vi "Model Initial Values - Main On Save Action.vi"(8 "error in (no error)":errorcluster, 11 "Device Item Ref in":T1 format="%.0x") -> (0 "error out":errorcluster, 3 "Device Item Ref out":T1 format="%.0x")   [LabVIEW 2011, in "Model Initial Values Custom Device.lvlib"]
uses:
  Model Initial Values Custom Device.lvlib
  <vilib>/NI Veristand/Custom Device API/Custom Device Item Ref.ctl
  Model Initial Values - Global.vi
  <vilib>/NI Veristand/Custom Device API/Custom Device API.lvlib
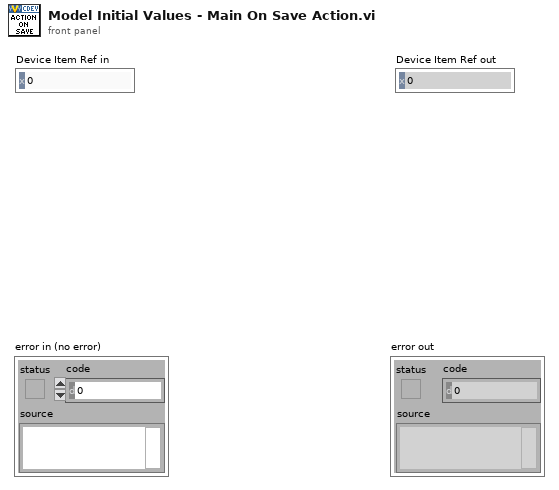
[diagram p1: front panel]
types:
  T1 = typedef "Custom Device API.lvlib/Custom Device Item Ref.ctl" = u64
  T2 = cluster{"Name":string, "Is Channel":bool, "GUID":string}
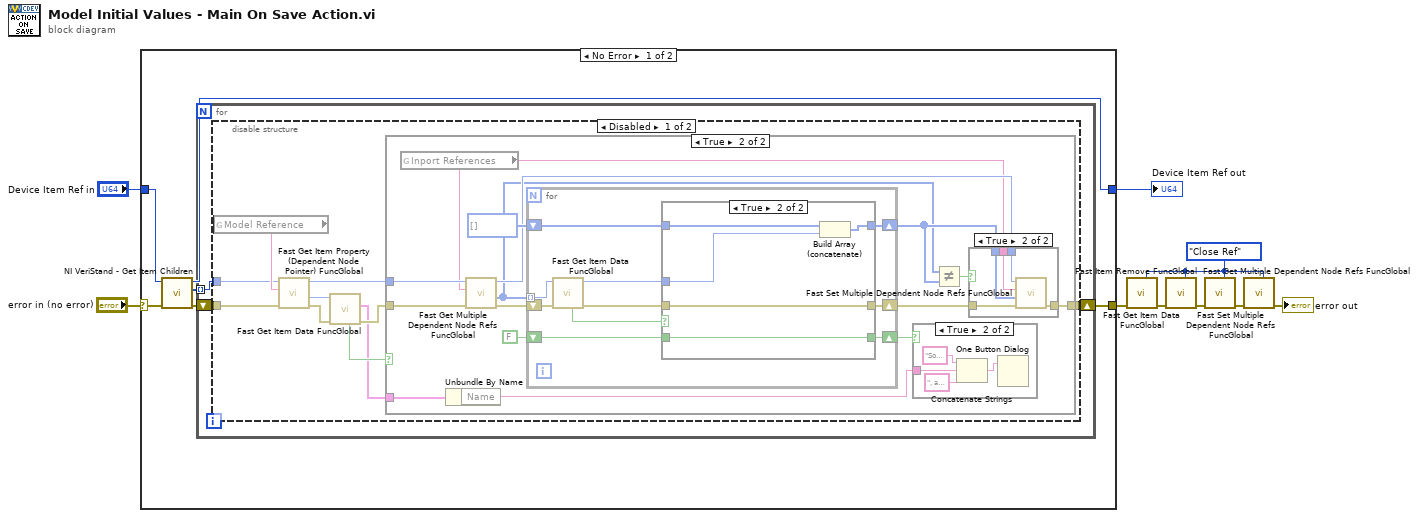
[diagram p0: block diagram]
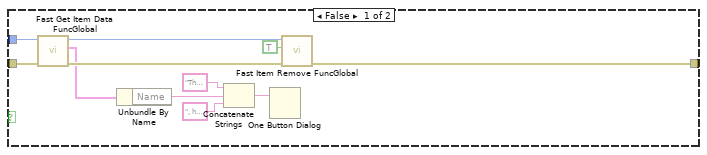
[diagram p2: hidden frame]
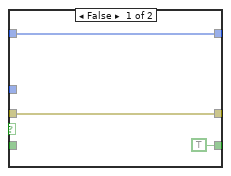
[diagram p5: hidden frame]
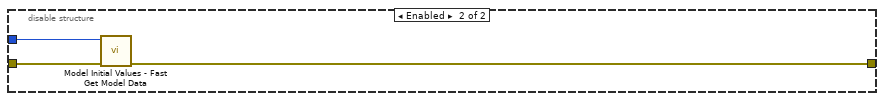
[diagram p6: hidden frame]
diagram:
  w1 = enum16{"Open or Add", "Close Ref"}."Close Ref" ("Action")
  n1 = case shown="No Error" "error in (no error)" {
    selector: "error in (no error)" -> [w14 w87]
    tunnel: [w15 w87] -> w6
    tunnel: "Device Item Ref in" -> [w12 w86]
    tunnel: [w10 w86] -> w7
    frame No Error {
      n2 = call <vilib>:"NI VeriStand - Get Item Children.vi"("error in (no error)"=w14, "Item Ref in"=w12) -> ("error out"=w13:errorcluster, "Child Refs"=w11:T1[], "Item Ref out"=w10:T1)  [unwired: 6 in, 1 out]
      n3 = for {
        shift-right: [w18] -> w15
        shift-left: w13 -> [w17]
        tunnel: w11 -> [w16] mode=indexing
        n4 = disable-structure shown="Disabled" {
          disable-tunnel: [w21 w83] -> w18
          disable-tunnel: w17 -> [w20 w85]
          disable-tunnel: w16 -> [w19 w84]
          frame Disabled {
            # "Initialization code."
            n5 = global read "Model Initial Values - Global.vi" "Model Reference"() -> (w23:string)
            n6 = call "Fast Get Item Property (Dependent Node Pointer) FuncGlobal.vi"("error in (no error)"=w20, "Property Name"=w23, "Item Ref in"=w19) -> ("error out"=w24:errorcluster, "Dependent Node Ref"=w26:T1, "Item Ref out"=w28:T1)  [unwired: 5 in, 1 out]
            n7 = call "Fast Get Item Data FuncGlobal.vi"("error in (no error)"=w24, "Item Ref in"=w26) -> ("error out"=w25:errorcluster, "Item Info"=w22:T2, "Found"=w27:bool)  [unwired: 6 in, 1 out]
            n8 = case shown="True" w27 {
              tunnel: [w34 w47] -> w21
              tunnel: w28 -> [w32 w53]
              tunnel: w25 -> [w33 w52]
              tunnel: w22 -> [_ w44]
              frame False {
                n9 = call "Fast Get Item Data FuncGlobal.vi"("error in (no error)"=w33, "Item Ref in"=w32) -> ("error out"=w30:errorcluster, "Item Info"=w29:T2, "Item Ref out"=w31:T1)  [unwired: 6 in, 1 out]
                n10 = Unbundle By Name(w29) -> ("Name"=w35:string)
                n11 = Concatenate Strings("The model, " ("message"), w35, ", has been deleted from the project and will therefore be removed from this custom device." ("message")) -> (w38:string)
                n12 = One Button Dialog(message=w38) -> ()  [unwired: 1 in, 1 out]
                n13 = call "Fast Item Remove FuncGlobal.vi"("error in (no error)"=w30, "Force Delete (F)"=TRUE, "Item Ref in"=w31) -> ("error out"=w34:errorcluster)  [unwired: 7 in, 1 out]
              }
              frame True {
                n14 = global read "Model Initial Values - Global.vi" "Inport References"() -> (w46:string)
                n15 = Unbundle By Name(w44) -> ("Name"=w45:string)
                n16 = call "Fast Get Multiple Dependent Node Refs FuncGlobal.vi"("error in (no error)"=w52, "Base Property Name"=w46, "Item Ref in"=w53) -> ("error out"=w54:errorcluster, "Dependent Node Refs"=w41:T1[], "Item Ref out"=w48:T1)  [unwired: 6 in]
                n17 = for {
                  tunnel: w41 -> [w73] mode=indexing
                  shift-right: [w70] -> w43
                  shift-left: w54 -> [w74]
                  shift-right: [w67] -> w42
                  shift-left: T1[] [] -> [w68]
                  shift-right: [w66] -> w49
                  shift-left: FALSE -> [w65]
                  n18 = call "Fast Get Item Data FuncGlobal.vi"("error in (no error)"=w74, "Item Ref in"=w73) -> ("error out"=w71:errorcluster, "Item Ref out"=w72:T1, "Found"=w69:bool)  [unwired: 6 in, 1 out]
                  n19 = case shown="True" w69 {
                    tunnel: w72 -> [_ w79]
                    tunnel: w71 -> [w76 w78]
                    tunnel: [w76 w78] -> w70
                    tunnel: w68 -> [w77 w82]
                    tunnel: [w77 w81] -> w67
                    tunnel: [TRUE w80] -> w66
                    tunnel: w65 -> [_ w80]
                    frame False {
                    }
                    frame True {
                      n20 = Build Array (concatenate)(w82, w79) -> (w81:T1[])
                    }
                  }
                }
                n21 = case shown="True" w49 {
                  tunnel: w45 -> [_ w61]
                  frame False {
                  }
                  frame True {
                    n22 = Concatenate Strings("Some inports have been deleted from the model, " ("message"), w61, ", and will therefore be removed from the \"Model Initial Values\" custom device." ("message")) -> (w64:string)
                    n23 = One Button Dialog(message=w64) -> ()  [unwired: 1 in, 1 out]
                  }
                }
                n24 = Not Equal?(x=w41, y=w42) -> (x != y?=w40:bool)
                n25 = case shown="True" w40 {
                  tunnel: w48 -> [_ w60]
                  tunnel: [w55 w59] -> w47
                  tunnel: w46 -> [_ w58]
                  tunnel: w43 -> [w55 w57]
                  tunnel: w42 -> [_ w56]
                  frame False {
                  }
                  frame True {
                    n26 = call "Fast Set Multiple Dependent Node Refs FuncGlobal.vi"("error in (no error)"=w57, "Dependent Node Refs"=w56, "Base Property Name"=w58, "Item Ref in"=w60) -> ("error out"=w59:errorcluster)  [unwired: 6 in, 1 out]
                  }
                }
              }
            }
          }
          frame Enabled {
            n27 = call "Model Initial Values - Fast Get Model Data.vi"("error in (no error)"=w85, "Local Model Ref in"=w84) -> ("error out"=w83:errorcluster)  [unwired: 4 in, 5 out]
          }
        }
      }
    }
    frame Error {
    }
  }
  "Device Item Ref out" <- w7
  n28 = call "Fast Get Item Data FuncGlobal.vi"("Action"=w1, "error in (no error)"=w6) -> ("error out"=w5:errorcluster)  [unwired: 6 in, 3 out]
  n29 = call "Fast Item Remove FuncGlobal.vi"("Action"=w1, "error in (no error)"=w5) -> ("error out"=w4:errorcluster)  [unwired: 8 in, 1 out]
  n30 = call "Fast Get Multiple Dependent Node Refs FuncGlobal.vi"("Action"=w1, "error in (no error)"=w4) -> ("error out"=w3:errorcluster)  [unwired: 7 in, 2 out]
  n31 = call "Fast Set Multiple Dependent Node Refs FuncGlobal.vi"("Action"=w1, "error in (no error)"=w3) -> ("error out"=→"error out":errorcluster)  [unwired: 8 in, 1 out]
